vi "ma_resample single-shot (spline).vi"(6 "#elements":i32, 8 "error in":errorcluster, 9 "t0":timestamp format="%<%.4X>T", 10 "dt":dbl=1.0 format="%.2p", 11 "waveform in":waveform(dbl)) -> (0 "error out":errorcluster, 1 "used t0":timestamp format="%<%.4X>T", 3 "resampled waveform out":waveform(dbl), 4 "t0 adjusted warning":bool)   [LabVIEW 2020, in "NI_MAPro.lvlib"]
doc: "This VI re-samples an unevenly sampled input signal to an evenly sampled waveform according to specified t0 and dt. If the specified t0 value is less than the first value of input X-array (that is the timestamp of the first input sample), then the VI will coerce t0 to the first valid value (greater than X(0)) that also fulfill the relation:\n\nT0_adjusted - t0_in = n * dt_in\n\nThis guarranty that any later comparison of waveforms will be correct with repsect to absolute time."
uses:
  NI_MAPro.lvlib
  NI_AALPro.lvlib
  NI_AALBase.lvlib
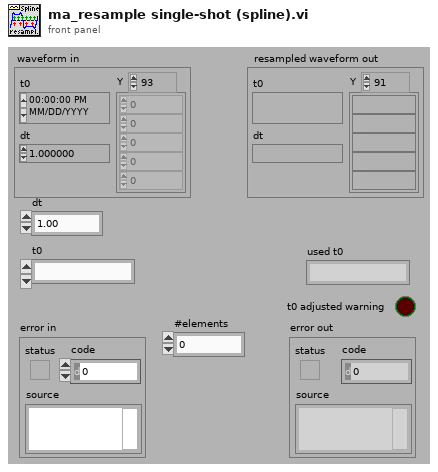
[diagram p1: front panel]
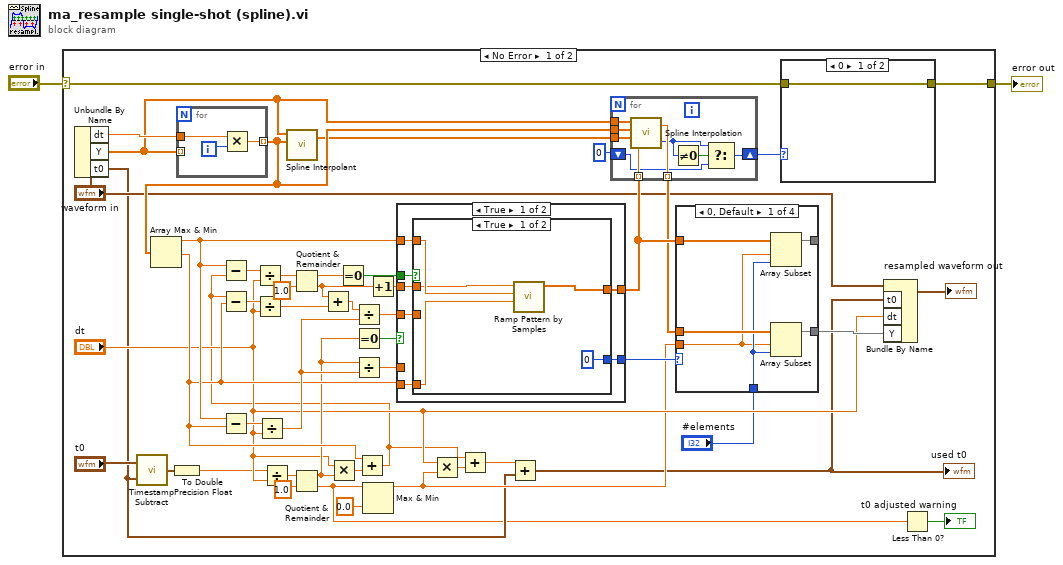
[diagram p0: block diagram]
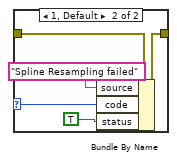
[diagram p2: hidden frame]
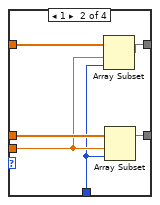
[diagram p3: hidden frame]
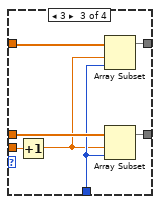
[diagram p4: hidden frame]
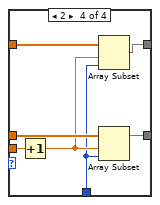
[diagram p5: hidden frame]
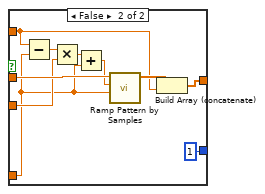
[diagram p6: hidden frame]
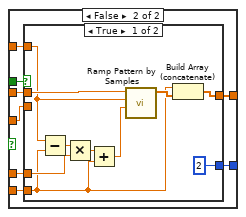
[diagram p7: hidden frame]
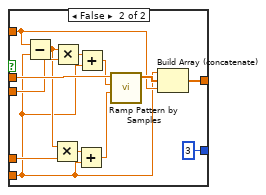
[diagram p8: hidden frame]
diagram:
  n1 = case shown="No Error" "error in" {
    selector: "error in" -> [w20 w149]
    tunnel: [w21 w149] -> w1
    frame No Error {
      n2 = Unbundle By Name("waveform in") -> ("dt"=w18:dbl, "Y"=w10:dbl[], "t0"=w4:timestamp)
      n3 = call "Timestamp Subtract.vi"("y"=w4, "x"="t0") -> ("x - y"=w30:timestamp)
      n4 = To Double Precision Float(number=w30) -> (double precision float=w7:dbl)
      n5 = for {
        tunnel: w18 -> [w69]
        tunnel: [w67] -> w13 mode=indexing
        tunnel: w10 -> [_] mode=indexing
        i -> [w68]
        n6 = Multiply(x=w69, y=w68) -> (x*y=w67:dbl)
      }
      n7 = Array Max & Min(array=w13) -> (max value=w40:dbl, min value=w28:dbl)  [unwired: 2 out]
      n8 = Subtract(x=w40, y=w28) -> (x-y=w39:dbl)
      n9 = Divide(x=w39, y="dt") -> (x/y=w37:dbl)
      n10 = Divide(x=w7, y="dt") -> (x/y=w32:dbl)
      n11 = call "Spline Interpolant.vi"("X"=w13, "Y"=w10) -> ("Interpolant"=w11:dbl[])  [unwired: 2 in, 1 out]
      n12 = Quotient & Remainder(x=w32, y=1.0) -> (x-y*floor(x/y)=w27:dbl, floor(x/y)=w3:dbl)
      n13 = Multiply(x="dt", y=w27) -> (x*y=w29:dbl)
      n14 = Equal To 0?(x=w27) -> (x = 0?=w46:bool)
      n15 = Divide(x=w27, y=w37) -> (x/y=w44:dbl)
      n16 = Add(x=w28, y=w29) -> (x+y=w24:dbl)
      n17 = Subtract(x=w40, y=w24) -> (x-y=w50:dbl)
      n18 = Subtract(x=w24, y=w28) -> (x-y=w51:dbl)
      n19 = Divide(x=w50, y="dt") -> (x/y=w38:dbl)
      n20 = Divide(x=w51, y="dt") -> (x/y=w34:dbl)
      n21 = Quotient & Remainder(x=w38, y=1.0) -> (x-y*floor(x/y)=w48:dbl, floor(x/y)=w36:dbl)
      n22 = Add(x=w36, y=w34) -> (x+y=w35:dbl)
      n23 = Equal To 0?(x=w48) -> (x = 0?=w47:bool)
      n24 = Divide(x=w35, y=w37) -> (x/y=w45:dbl)
      n25 = Max & Min(x=w3, y=0.0) -> (max(x,y)=w23:dbl)  [unwired: 1 out]
      n26 = Increment(x=w36) -> (x+1=w41:dbl)
      n27 = case shown="True" w46 {
        tunnel: w47 -> [w102 w125]
        tunnel: w28 -> [w101 w124]
        tunnel: w40 -> [w100 w123]
        tunnel: [w99 w122] -> w15
        tunnel: w41 -> [w98 w121]
        tunnel: w45 -> [w97 w120]
        tunnel: w44 -> [_ w119]
        tunnel: [w96 w118] -> w42
        frame True {
          n28 = case shown="True" w102 {
            tunnel: w101 -> [w107 w109]
            tunnel: w100 -> [w106 w114]
            tunnel: [w105 w116] -> w99
            tunnel: w98 -> [w104 w117]
            tunnel: w97 -> [_ w112]
            tunnel: [0 1] -> w96
            frame True {
              n29 = call "Ramp Pattern by Samples.vi"("start"=w107, "end"=w106, "samples"=w104) -> ("Ramp Pattern"=w105:dbl[])  [unwired: 7 in, 1 out]
            }
            frame False {
              n30 = Subtract(x=w114, y=w109) -> (x-y=w113:dbl)
              n31 = Multiply(x=w113, y=w112) -> (x*y=w110:dbl)
              n32 = Add(x=w110, y=w109) -> (x+y=w111:dbl)
              n33 = call "Ramp Pattern by Samples.vi"("start"=w109, "end"=w111, "samples"=w117) -> ("Ramp Pattern"=w115:dbl[])  [unwired: 7 in, 1 out]
              n34 = Build Array (concatenate)(w115, w114) -> (w116:dbl[])
            }
          }
        }
        frame False {
          n35 = case shown="True" w125 {
            tunnel: w124 -> [w127 w138]
            tunnel: w123 -> [w132 w145]
            tunnel: [w129 w147] -> w122
            tunnel: w121 -> [w135 w148]
            tunnel: w120 -> [_ w144]
            tunnel: w119 -> [w131 w140]
            tunnel: [2 3] -> w118
            frame True {
              n36 = Subtract(x=w132, y=w127) -> (x-y=w134:dbl)
              n37 = Multiply(x=w134, y=w131) -> (x*y=w133:dbl)
              n38 = Add(x=w133, y=w127) -> (x+y=w130:dbl)
              n39 = call "Ramp Pattern by Samples.vi"("start"=w130, "end"=w132, "samples"=w135) -> ("Ramp Pattern"=w128:dbl[])  [unwired: 7 in, 1 out]
              n40 = Build Array (concatenate)(w127, w128) -> (w129:dbl[])
            }
            frame False {
              n41 = Subtract(x=w145, y=w138) -> (x-y=w139:dbl)
              n42 = Multiply(x=w139, y=w140) -> (x*y=w141:dbl)
              n43 = Multiply(x=w139, y=w144) -> (x*y=w142:dbl)
              n44 = Add(x=w141, y=w138) -> (x+y=w137:dbl)
              n45 = Add(x=w142, y=w138) -> (x+y=w143:dbl)
              n46 = call "Ramp Pattern by Samples.vi"("start"=w137, "end"=w143, "samples"=w148) -> ("Ramp Pattern"=w146:dbl[])  [unwired: 7 in, 1 out]
              n47 = Build Array (concatenate)(w138, w146, w145) -> (w147:dbl[])
            }
          }
        }
      }
      n48 = Multiply(x="dt", y=w23) -> (x*y=w25:dbl)
      n49 = Add(x=w24, y=w25) -> (x+y=w6:dbl)
      n50 = Add(x=w6, y=w4) -> (x+y=w5:timestamp)
      "used t0" <- w5
      n51 = for {
        tunnel: w11 -> [w60]
        tunnel: w10 -> [w59]
        tunnel: w15 -> [w58] mode=indexing
        tunnel: [w57] -> w14 mode=indexing
        tunnel: w13 -> [w54]
        shift-right: [w52] -> w12
        shift-left: 0 -> [w53]
        n52 = call "Spline Interpolation.vi"("x value"=w58, "Interpolant"=w60, "X"=w54, "Y"=w59) -> ("error"=w55:i32, "interpolation value"=w57:dbl)
        n53 = Not Equal To 0?(x=w55) -> (x != 0?=w56:bool)
        n54 = Select(t=w55, s=w56, f=w53) -> (s? t:f=w52:i32)
      }
      n55 = case shown="0, Default" w42 {
        tunnel: w14 -> [w73 w80 w85 w94]
        tunnel: [w74 w81 w88 w95] -> w33
        tunnel: w15 -> [w72 w78 w87 w91]
        tunnel: [w75 w79 w86 w92] -> _
        tunnel: w23 -> [w70 w77 w84 w90]
        tunnel: "#elements" -> [w71 w76 w83 w89]
        frame 0, Default {
          n56 = Array Subset(array=w72, index=w70, length=w71) -> (w75:dbl[])
          n57 = Array Subset(array=w73, index=w70, length=w71) -> (w74:dbl[])
        }
        frame 1 {
          n58 = Array Subset(array=w78, index=w77, length=w76) -> (w79:dbl[])
          n59 = Array Subset(array=w80, index=w77, length=w76) -> (w81:dbl[])
        }
        frame 3 {
          n60 = Increment(x=w84) -> (x+1=w82:dbl)
          n61 = Array Subset(array=w87, index=w82, length=w83) -> (w86:dbl[])
          n62 = Array Subset(array=w85, index=w82, length=w83) -> (w88:dbl[])
        }
        frame 2 {
          n63 = Increment(x=w90) -> (x+1=w93:dbl)
          n64 = Array Subset(array=w91, index=w93, length=w89) -> (w92:dbl[])
          n65 = Array Subset(array=w94, index=w93, length=w89) -> (w95:dbl[])
        }
      }
      n66 = case shown="0" w12 {
        selector: w12 -> [_ w64]
        tunnel: w20 -> [w61 w66]
        tunnel: [w61 w65] -> w21
        frame 0 {
        }
        frame 1, Default {
          n67 = Bundle By Name(cluster=w66, "source"="Spline Resampling failed", "code"=w64, "status"=TRUE) -> (w65:errorcluster)
        }
      }
      n68 = Bundle By Name(cluster="waveform in", "t0"=w5, "dt"="dt", "Y"=w33) -> (→"resampled waveform out":waveform(dbl))
      n69 = Less Than 0?(x=w3) -> (x < 0?=→"t0 adjusted warning":bool)
    }
    frame Error {
    }
  }
  "error out" <- w1
